vi "Digio Port Config_DAQmx.vi"(6 "error in":errorcluster, 8 "DO Task":refnum<k21>="BlueSimple_DO", 9 "DI Task":refnum<k21>="BlueSimple_DI") -> (0 "error out":errorcluster)   [LabVIEW 2010]
uses:
  Controls/Bits to Write.ctl
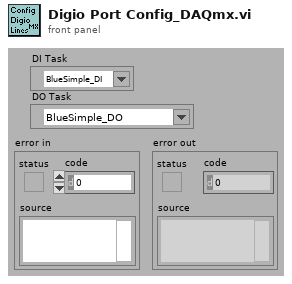
[diagram p1: front panel]
types:
  T1 = typedef "Bits to Write.ctl" = enum16{"LED 1 on", "LED 1 off", "LED 2 on", "LED 2 off", "LED 3 on", "LED 3 off", "LED 4 on", "LED 4 off", "All LEDs on", "All LEDs off", "In trial on", "In trial off", "Buzzer on", "Buzzer off", "Reward on", "Reward off", "Target number", "Trial type preQ on", "Trial type preQ off", "Error on", "Error off", "Trial number", "DBS on", "DBS off", "Sine on", "Sine off", "All Bits On", "All Bits Off", "Init", "Specify mask/pattern"}
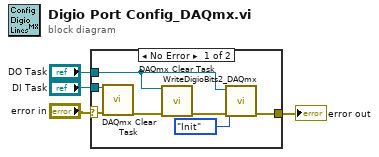
[diagram p0: block diagram]
diagram:
  n1 = case shown="No Error" "error in" {
    selector: "error in" -> [w9 w12]
    tunnel: "DI Task" -> [w11 _]
    tunnel: "DO Task" -> [w6 _]
    tunnel: [w7 w12] -> w2
    frame No Error {
      n2 = call <vilib>:"DAQmx Clear Task.vi"("task in"=w11, "error in"=w9) -> ("error out"=w10:errorcluster)  [unwired: 13 in]
      n3 = call <vilib>:"DAQmx Clear Task.vi"("task in"=w6, "error in"=w10) -> ("error out"=w8:errorcluster)  [unwired: 13 in]
      n4 = call "WriteDigioBits2_DAQmx.vi"("error in"=w8, "Bits to write"=Bits_to_Write."Init", "DO Task"=w6) -> ("error out"=w7:errorcluster)  [unwired: 8 in]
    }
    frame Error {
    }
  }
  "error out" <- w2
